vi "Select QCh & dt.vi"(7 "Quench Channel in":i32, 8 "Error In":errorcluster, 9 "Stop Time in":dbl[unit]=0.1, 10 "Start Time in":dbl[unit]=-0.1, 11 "KIT-QA in":refnum<class "KIT-QA.lvclass">) -> (0 "Error Out":errorcluster, 1 "Stop Time out":dbl[unit]=0.1, 2 "Start Time out":dbl[unit]=-0.1, 3 "OK":bool, 5 "Quench Channel out":i32)   [LabVIEW 2016, in "KIT-QA.lvlib" / "KIT-QA.lvclass"]
doc: "User can override the default quench channel selection and time frame to save to TDMS."
uses:
  KIT-QA.lvclass
  KIT-QA.lvclass/KIT-QA.ctl
panel:
  in  "OK":bool
  in  "Cancel":bool
  in  "Stop Time":dbl[unit]=0.1
  in  "Start Time":dbl[unit]=-0.1
  in  "Channel List":i32(listbox)
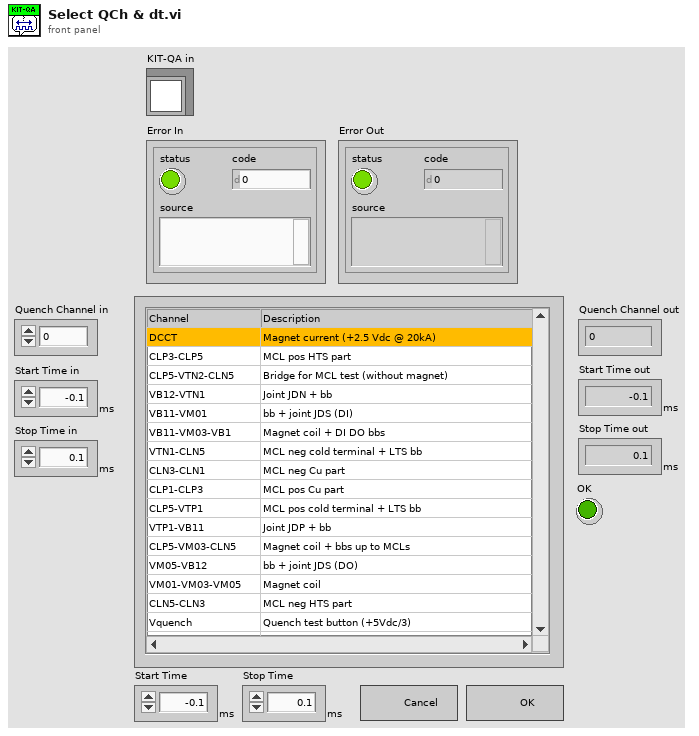
[diagram p1: front panel]
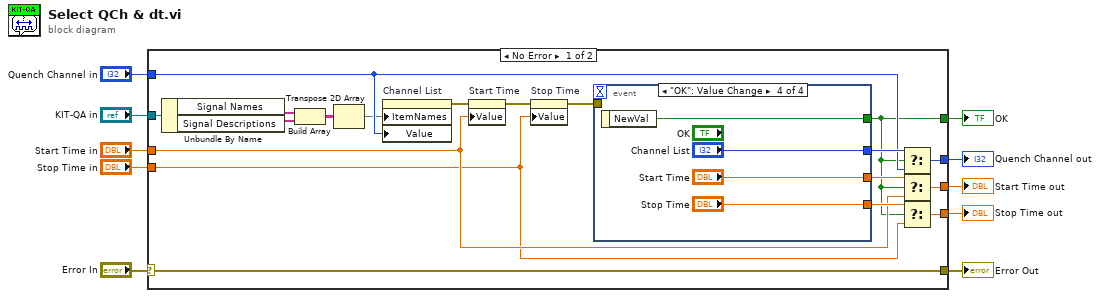
[diagram p0: block diagram]
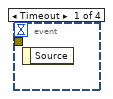
[diagram p2: hidden frame]
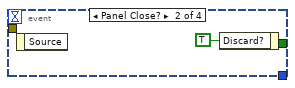
[diagram p3: hidden frame]
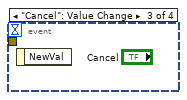
[diagram p4: hidden frame]
diagram:
  n1 = case shown="No Error" "Error In" {
    selector: "Error In" -> [w13 w38]
    tunnel: "KIT-QA in" -> [w26 _]
    tunnel: [w19 w35] -> w9
    tunnel: [w18 w36] -> w8
    tunnel: [w17 w37] -> w7
    tunnel: "Quench Channel in" -> [w16 w35]
    tunnel: "Start Time in" -> [w15 w36]
    tunnel: "Stop Time in" -> [w14 w37]
    tunnel: [w13 w38] -> w2
    tunnel: [w12 _] -> w1
    frame No Error {
      n2 = Unbundle By Name(w26) -> ("Signal Names"=w29:string[], "Signal Descriptions"=w28:string[])
      n3 = Build Array(w29, w28) -> (w27:string[][])
      n4 = Transpose 2D Array(2D array=w27) -> (transposed array=w11:string[][])
      n5 = property on="Channel List" class="MCListbox (strict)"("ItemNames"=w11, "Value"=w16) -> (error out=w25:errorcluster)  [unwired: 2 in, 1 out]
      n6 = property on="Start Time" class="DigNum (strict)"(error in=w25, "Value"=w15) -> (error out=w24:errorcluster)  [unwired: 1 in, 1 out]
      n7 = property on="Stop Time" class="DigNum (strict)"(error in=w24, "Value"=w14) -> (error out=w23:errorcluster)  [unwired: 1 in, 1 out]
      n8 = event shown="[3] \"OK\": Value Change" {
        selector: _ -> [_ _ _ _]
        dyn-events: _ -> [_ _ _ _]
        timeout: _ -> [_ _ _ _]
        tunnel: [_ _ _ w34] -> w12
        tunnel: w23 -> [_ _ _ _]
        tunnel: [_ _ _ "Channel List"] -> w22
        tunnel: [_ _ _ "Start Time"] -> w21
        tunnel: [_ _ _ "Stop Time"] -> w20
        event Timeout {
          n9 = event-data() -> ()  [unwired: 1 in, 1 out]
        }
        event Panel Close? {
          n10 = event-data() -> ()  [unwired: 1 in, 1 out]
          n11 = event-data("Discard?"=TRUE) -> ()  [unwired: 1 in, 1 out]
        }
        event "Cancel": Value Change {
          n12 = event-data() -> ()  [unwired: 1 in, 1 out]
        }
        event "OK": Value Change {
          n13 = event-data() -> ("NewVal"=w34:bool)  [unwired: 1 in]
        }
      }
      n14 = Select(t=w22, s=w12, f=w16) -> (s? t:f=w19:i32)
      n15 = Select(t=w21, s=w12, f=w15) -> (s? t:f=w18:dbl[unit])
      n16 = Select(t=w20, s=w12, f=w14) -> (s? t:f=w17:dbl[unit])
    }
    frame Error {
    }
  }
  "Error Out" <- w2
  "Quench Channel out" <- w9
  "Start Time out" <- w8
  "Stop Time out" <- w7
  "OK" <- w1
